vi "Enable TREADY.vi"(10 "m_axis_tready":refnum<k21>, 11 "niInstr AXI4-Stream Reader v1 FPGA in":refnum<class "niInstr AXI4-Stream Reader v1 FPGA.lvclass">) -> (3 "niInstr AXI4-Stream Reader v1 FPGA out":refnum<class "niInstr AXI4-Stream Reader v1 FPGA.lvclass">)   [LabVIEW 2015, in "niInstr AXI4-Stream Reader v1 FPGA.lvclass"]
doc: "Enables TREADY compilation as part of the AXI4-Stream Reader interface.\n\n<B>Input Parameters</B>\n\n<B>m_axis_tready</B> specifies the FPGA resource to use for TREADY.\n\n<B>niInstr AXI4-Stream Reader v1 FPGA in</B> takes in a reference to the AXI4-Stream Reader from the previous VI\n\n<B>Output Parameters</B>\n\n<B>niInstr AXI4-Stream Reader v1 FPGA out</B> passes a reference to the AXI4-Stream Reader to the next VI."
uses:
  <instrlib>/_niInstr/CLIP Adapters/v1/FPGA/AXI4-Stream/Reader/niInstr AXI4-Stream Reader v1 FPGA.lvclass
  <instrlib>/_niInstr/CLIP Adapters/v1/FPGA/AXI4-Stream/Reader/niInstr AXI4-Stream Reader v1 FPGA.lvclass/niInstr AXI4-Stream Reader v1 FPGA.ctl
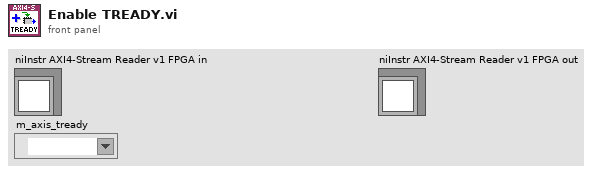
[diagram p1: front panel]
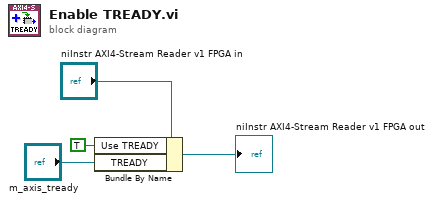
[diagram p0: block diagram]
diagram:
  n1 = Bundle By Name(cluster="niInstr AXI4-Stream Reader v1 FPGA in", "Use TREADY"=TRUE, "TREADY"="m_axis_tready") -> (→"niInstr AXI4-Stream Reader v1 FPGA out":refnum<class "niInstr AXI4-Stream Reader v1 FPGA.lvclass">)
